vi "NetworkScan2.vi"() -> ()   [LabVIEW 2013]
uses:
  Global 1.vi
panel:
  in  "Adj Phase Display":bool=TRUE
  in  "Phase offset":dbl=9.0 format="%#_13g"
  in  "Phase reverse":bool
  in  "dB Adjust":dbl format="%#_13g"
  in  "Phase Slope":dbl=0.22 format="%#_13g"
  out "Freq":dbl[](array[numeric])=[50.0, 70.0, 90.0, 110.0, 130.0, 150.0, 170.0, 190.0, 210.0, 230.0, 250.0, 270.0, 290.0, 310.0, 330.0, 350.0, 370.0, 390.0, 410.0, 430.0, 450.0, 470.0, 490.0, 510.0, 530.0, 550.0, 570.0, 590.0]
  out "R":dbl[](array[numeric])=[51.39705226143004, 51.825157289879385, 52.29490017086176, 52.52103640128099, 52.80870403757797, 53.163512769280565, 53.42736324449612, 53.69682438236105, 54.65427148956741, 54.05801308215068, 54.56869132407272, 54.39339711204505, 54.48165615139422, 54.755961052429505, 54.94039884901909, 55.2541002690093, 55.69359971033443, 56.03821438031888, 56.291069946254225, 56.42902418783239, 56.8327333797083, 57.12107510293691, 57.1090243248507, 57.40495313083003, 57.87411821297632, 58.20928162412048, 58.563028446653554, 58.9207886281663]
  out "X":dbl[](array[numeric])=[3.314384336838985, 3.116641722448325, 2.8997180220653047, 2.7163285312028536, 2.541197206109193, 1.9733873117266927, 1.66365666259649, 1.2201611621763202, 0.966829160353334, -0.010719208003959988, -0.17205219858295065, 0.039184975155916305, 0.04566213827065729, 0.14099681156751956, 0.3331888543010345, 0.2178736519480885, 0.2443683106774066, 0.4348294971509995, 0.40400408584390385, 0.24329114919378528, 0.26838154433644296, 0.1573331889074762, 0.4307366964870689, 0.45955661557684224, 0.5011201257734776, 0.4575689744142302, 0.3285854990698071, 0.43958854255272406]
  out "Z":dbl[](array[numeric])=[51.5038068951845, 51.918786424057, 52.375232204620225, 52.59123220988561, 52.86981090725445, 53.20012544582523, 53.453258990919686, 53.71068554777353, 54.662822381218575, 54.05801414491097, 54.56896255914131, 54.39341122646114, 54.481675286555046, 54.75614258579624, 54.94140916014012, 55.254529818522094, 55.69413581847039, 56.0399013884408, 56.292519707288506, 56.42954865470969, 56.83336706603217, 57.12129178027831, 57.11064868689629, 57.40679259665804, 57.87628772053382, 58.21108001542762, 58.563950253323526, 58.92242841780874]
  out "rho":dbl[](array[numeric])=[0.03545339823862092, 0.03545339823862092, 0.036135509333077416, 0.036135509333077416, 0.03683074400858102, 0.036135509333077416, 0.03683074400858102, 0.03753935475828268, 0.045420291648158743, 0.03899773883575112, 0.04372172572841054, 0.04208668045282904, 0.04289641359808358, 0.045420291648158743, 0.04718484595550288, 0.04996104067702601, 0.05391836595759612, 0.05709073793282292, 0.05930868290572584, 0.06044976140926764, 0.06400641832195533, 0.06649303382021261, 0.06649303382021261, 0.06907625301538464, 0.07314046314727217, 0.07598193145591736, 0.07893378930547613, 0.08200032527122701]
  out "Theta (rad)":dbl[](array[numeric])=[1.1392083305611427, 1.0104217312459167, 0.8729688371640744, 0.796180006448542, 0.7107248809663943, 0.5386068078180897, 0.4358190928027104, 0.30703249348748424, 0.19557848370548936, -0.0025384737426618997, -0.0359958306251161, 0.008543465391970878, 0.009751287575979536, 0.028291699293219123, 0.06416470054369075, 0.039373638427852395, 0.04058146061186093, 0.0677881670957166, 0.06032969451310942, 0.035538632397271064, 0.03674645458127959, 0.020621687232057196, 0.05649468848252858, 0.057702510666536616, 0.05891033285054589, 0.051451860267938465, 0.03532709291871557, 0.045201209869340064]
  out "Smith Chart":picture
  out "Handle":u32=147464592
  out "Device Description":string="DLP-IO20"
  in  "Device Index":u32
  in  "Phase adjust":bool=TRUE
  in  "Fstep":dbl=20.0 format="%#_13g"
  in  "Fmin":dbl=50.0 format="%#_13g"
  in  "Fmax (MHz)":dbl=600.0 format="%#_13g"
  out "Reflected Angle (deg)":cluster{"Fmin":dbl, "Fstep":dbl, dbl[]}(graph)={"Fmin"=50.0, "Fstep"=20.0, [65.27663734115347, 57.89716520039102, 50.02111436950146, 45.621114369501456, 40.72453567937439, 30.862170087976537, 24.972434017595305, 17.592961876832845, 11.20664711632454, -0.14545454545452685, -2.062561094819152, 0.4895405669599313, 0.5587487781036273, 1.6211143695014556, 3.67663734115348, 2.256109481915942, 2.325317693059631, 3.884261974584561, 3.4568914956011696, 2.0363636363636317, 2.1055718475073206, 1.1816226783968773, 3.2371456500488875, 3.306353861192548, 3.3755620723362796, 2.948191593352874, 2.024242424242402, 2.5900293255131857]}
  out "Reflected Power (dBc)":cluster{"Fmin":dbl, "Fstep":dbl, dbl[]}(graph)={"Fmin"=50.0, "Fstep"=20.0, [-29.006842619745846, -29.006842619745846, -28.841316389703486, -28.841316389703486, -28.67579015966113, -28.841316389703486, -28.67579015966113, -28.51026392961877, -26.85500162919518, -28.179211469534053, -27.1860540892799, -27.517106549364616, -27.351580319322256, -26.85500162919518, -26.523949169110463, -26.027370478983386, -25.36526555881395, -24.868686868686872, -24.537634408602152, -24.372108178559795, -23.875529488432715, -23.544477028347995, -23.544477028347995, -23.213424568263278, -22.7168458781362, -22.385793418051485, -22.054740957966764, -21.723688497882048]}
  # "Network Analyzer"
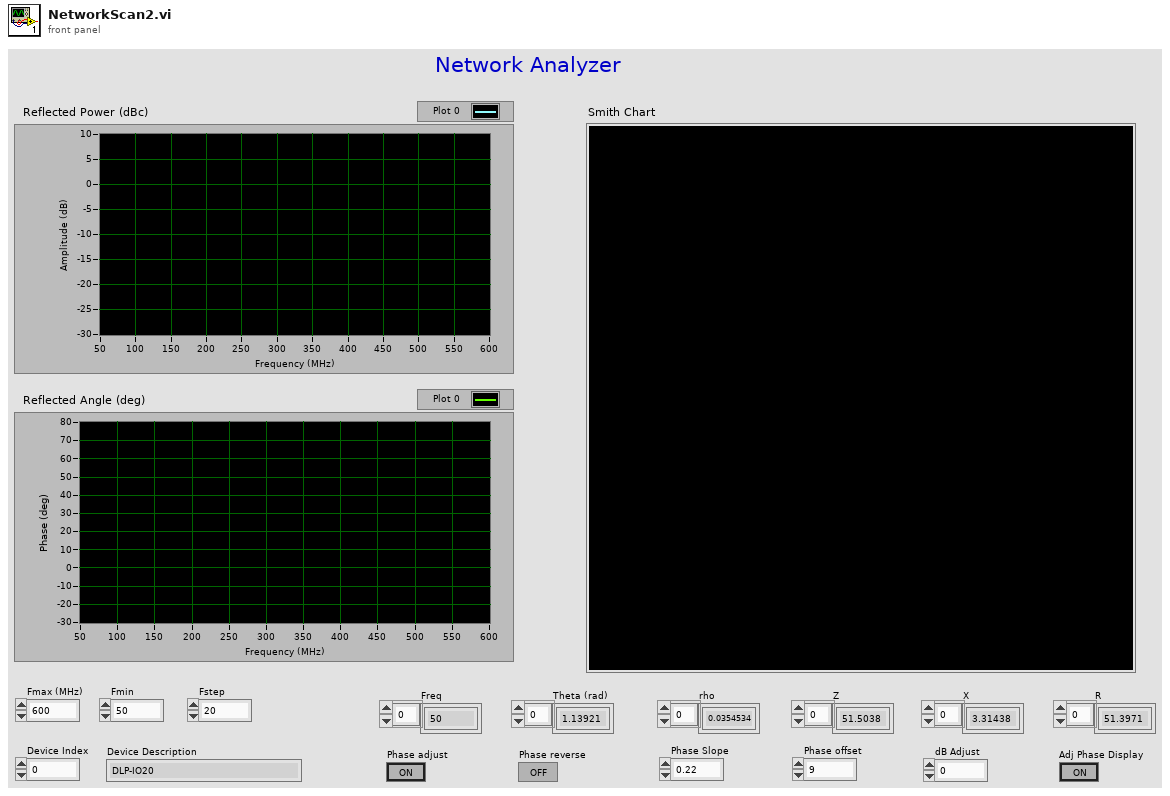
[diagram p1: front panel]
types:
  T1 = typedef "LVBoundsTypeDef.ctl" = cluster{"Width":u32, "Height":u32}
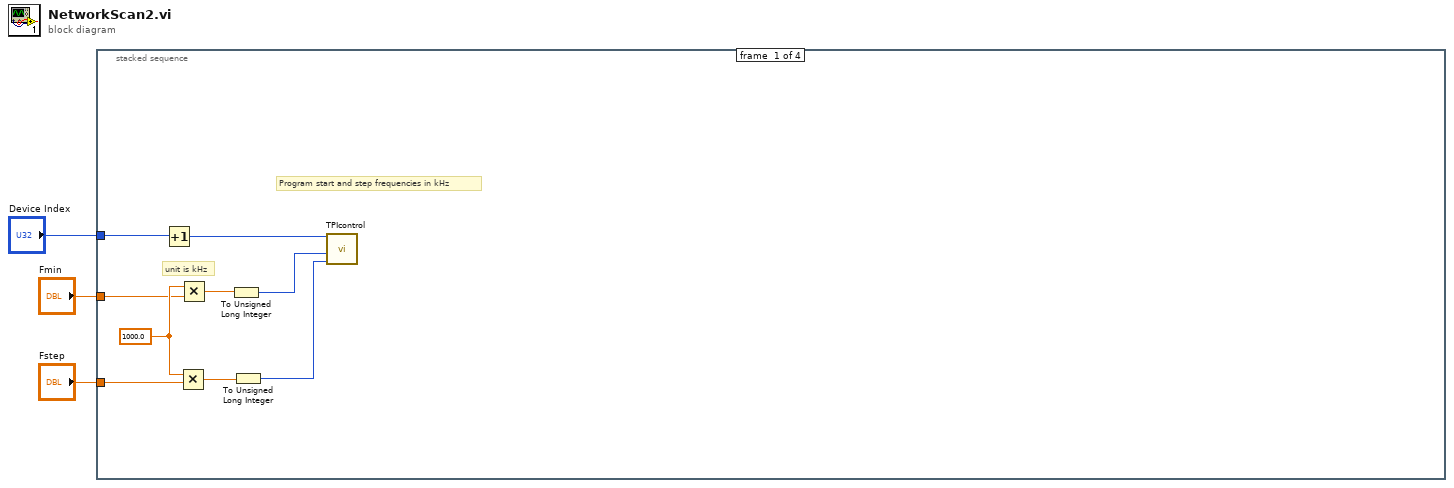
[diagram p0: block diagram]
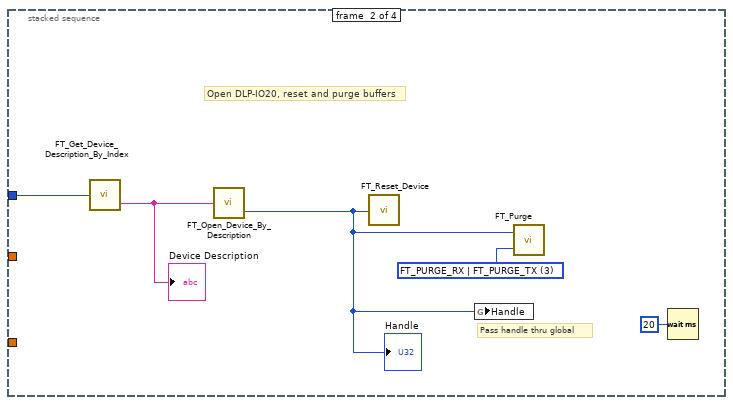
[diagram p2: hidden frame]
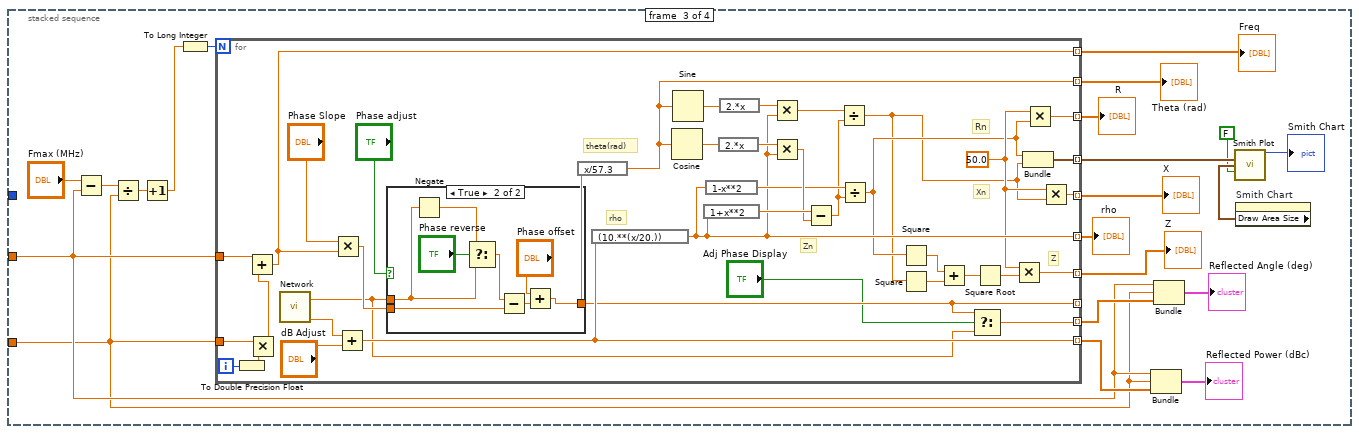
[diagram p3: hidden frame]
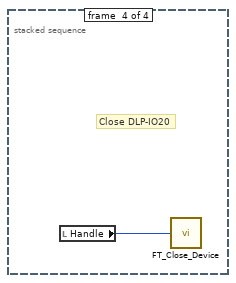
[diagram p5: hidden frame]
diagram:
  n1 = stacked-sequence {
    tunnel: "Fmin" -> [w10 _ w19 _]
    tunnel: "Fstep" -> [w11 _ w18 _]
    tunnel: "Device Index" -> [w5 w13 _ _]
    frame #0 {
      w12 = 1000.0
      # "unit is kHz"
      # "Program start and step frequencies in kHz"
      n2 = Increment(x=w5) -> (x+1=w4:u32)
      n3 = Multiply(x=w12, y=w11) -> (x*y=w8:dbl)
      n4 = Multiply(x=w12, y=w10) -> (x*y=w9:dbl)
      n5 = To Unsigned Long Integer(number=w9) -> (unsigned 32bit integer=w7:u32)
      n6 = To Unsigned Long Integer(number=w8) -> (unsigned 32bit integer=w6:u32)
      n7 = call "TPIcontrol.vi"("Fstep (kHz)"=w6, "Freq (kHz)"=w7, "Device index"=w4) -> ()  [unwired: 9 in]
    }
    frame #1 {
      w16 = u32 3 items=["FT_PURGE_RX"=1, "FT_PURGE_TX"=2, "FT_PURGE_RX | FT_PURGE_TX"=3] ("Purge Flags")
      # "Pass handle thru global"
      # "Open DLP-IO20, reset and purge buffers"
      n8 = call "FT_Get_Device_Description_By_Index.vi"("Device Index"=w13) -> ("Device Description"=w17:string)  [unwired: 1 out]
      "Device Description" <- w17
      n9 = call "FT_Open_Device_By_Description.vi"("Device Description"=w17) -> ("Handle"=w14:u32)  [unwired: 1 out]
      "Handle" <- w14
      n10 = call "FT_Reset_Device.vi"("Handle"=w14) -> ()  [unwired: 1 out]
      n11 = global write "Global 1.vi" "Handle"(w14) -> ()
      n12 = call "FT_Purge.vi"("Purge Flags"=w16, "Handle"=w14) -> ()  [unwired: 1 out]
      n13 = Wait (ms)(milliseconds to wait=u32 20) -> ()  [unwired: 1 out]
    }
    frame #2 {
      n14 = Subtract(x="Fmax (MHz)", y=w19) -> (x-y=w35:dbl)
      n15 = Divide(x=w35, y=w18) -> (x/y=w32:dbl)
      n16 = Increment(x=w32) -> (x+1=w33:dbl)
      n17 = To Long Integer(number=w33) -> (32bit integer=w34:i32)
      n18 = for {
        N: w34 -> [_]
        tunnel: [w66] -> w31 mode=indexing
        tunnel: [w40] -> _ mode=indexing
        tunnel: w19 -> [w71]
        tunnel: w18 -> [w73]
        tunnel: [w51] -> w30 mode=indexing
        tunnel: [w53] -> w29 mode=indexing
        tunnel: [w63] -> w28 mode=indexing
        tunnel: [w54] -> w27 mode=indexing
        tunnel: [w55] -> w26 mode=indexing
        tunnel: [w65] -> w23 mode=indexing
        tunnel: [w64] -> w21 mode=indexing
        tunnel: [w41] -> w20 mode=indexing
        i -> [w74]
        w52 = 50.0
        # "Xn"
        # "Rn"
        # "Zn"
        # "Z"
        # "rho"
        # "theta(rad)"
        n19 = To Double Precision Float(number=w74) -> (double precision float=w72:dbl)
        n20 = Multiply(x=w73, y=w72) -> (x*y=w70:dbl)
        n21 = Add(x=w71, y=w70) -> (x+y=w64:dbl)
        n22 = call "Network.vi"() -> ("dB refl"=w75:dbl, "deg refl"=w42:dbl)  [unwired: 2 out]
        n23 = Multiply(x="Phase Slope", y=w64) -> (x*y=w68:dbl)
        n24 = Add(x=w75, y="dB Adjust") -> (x+y=w66:dbl)
        n25 = case shown="True" "Phase adjust" {
          tunnel: w42 -> [w77 w79]
          tunnel: w68 -> [_ w85]
          tunnel: [w77 w83] -> w40
          frame False {
          }
          frame True {
            n26 = Negate(x=w79) -> (-x=w80:dbl)
            n27 = Select(t=w80, s="Phase reverse", f=w79) -> (s? t:f=w78:dbl)
            n28 = Subtract(x=w78, y=w85) -> (x-y=w84:dbl)
            n29 = Add(x="Phase offset", y=w84) -> (x+y=w83:dbl)
          }
        }
        n30 = expression code="x/57.3"(w40) -> (w63:dbl)
        n31 = expression code="(10.**(x/20.))"(w66) -> (w53:dbl)
        n32 = Cosine(x=w63) -> (cos(x)=w61:dbl)
        n33 = Sine(x=w63) -> (sin(x)=w62:dbl)
        n34 = expression code="1+x**2"(w53) -> (w58:dbl)
        n35 = expression code="1-x**2"(w53) -> (w56:dbl)
        n36 = expression code="2.*x"(w61) -> (w59:dbl)
        n37 = expression code="2.*x"(w62) -> (w60:dbl)
        n38 = Multiply(x=w60, y=w53) -> (x*y=w50:dbl)
        n39 = Multiply(x=w59, y=w53) -> (x*y=w57:dbl)
        n40 = Subtract(x=w58, y=w57) -> (x-y=w49:dbl)
        n41 = Divide(x=w50, y=w49) -> (x/y=w43:dbl)
        n42 = Divide(x=w56, y=w49) -> (x/y=w44:dbl)
        n43 = Square(x=w44) -> (x^2=w46:dbl)
        n44 = Square(x=w43) -> (x^2=w45:dbl)
        n45 = Add(x=w46, y=w45) -> (x+y=w47:dbl)
        n46 = Select(t=w40, s="Adj Phase Display", f=w42) -> (s? t:f=w41:dbl)
        n47 = Square Root(x=w47) -> (sqrt(x)=w48:dbl)
        n48 = Multiply(x=w52, y=w48) -> (x*y=w51:dbl)
        n49 = Bundle(w44, w43) -> (w65:cluster{dbl, dbl})  [unwired: 1 in]
        n50 = Multiply(x=w52, y=w44) -> (x*y=w55:dbl)
        n51 = Multiply(x=w52, y=w43) -> (x*y=w54:dbl)
      }
      "Z" <- w30
      "X" <- w27
      "R" <- w26
      "Theta (rad)" <- w28
      "rho" <- w29
      "Freq" <- w21
      n52 = Bundle("Fmin"=w19, "Fstep"=w18, w31) -> (→"Reflected Power (dBc)":cluster{"Fmin":dbl, "Fstep":dbl, dbl[]})  [unwired: 1 in]
      n53 = Bundle("Fmin"=w19, "Fstep"=w18, w20) -> (→"Reflected Angle (deg)":cluster{"Fmin":dbl, "Fstep":dbl, dbl[]})  [unwired: 1 in]
      n54 = property on="Smith Chart" class="Pict"() -> ("Draw Area Size"=w24:T1)  [unwired: 2 in, 2 out]
      n55 = call <vilib>:"Smith Plot.vi"("smith plot"=w23, "dimensions (w,h)"=w24, "dimensions incl scales? (T)"=FALSE) -> ("new picture"=→"Smith Chart":picture)  [unwired: 12 in]
    }
    frame #3 {
      # "Close DLP-IO20"
      n56 = local read "Handle"() -> (w86:u32)
      n57 = call "FT_Close_Device.vi"("Handle"=w86) -> ()  [unwired: 1 out]
    }
  }
